vi "Set Object Size Difference.vi"(8 "error in (no error)":errorcluster, 9 "dSize":cluster{"width":i32, "height":i32}, 11 "GObj Refnum":refnum<vi>) -> (0 "error out":errorcluster, 2 "dSize":cluster{"width":i32, "height":i32})   [LabVIEW 2013, in "IObject.lvclass"]
uses:
  IObject.lvclass
  <vilib>/Utility/error.llb/Error Cluster From Error Code.vi
  <vilib>/ErrorRing/Error Ring.xnode
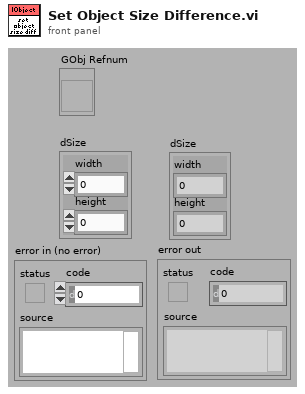
[diagram p1: front panel]
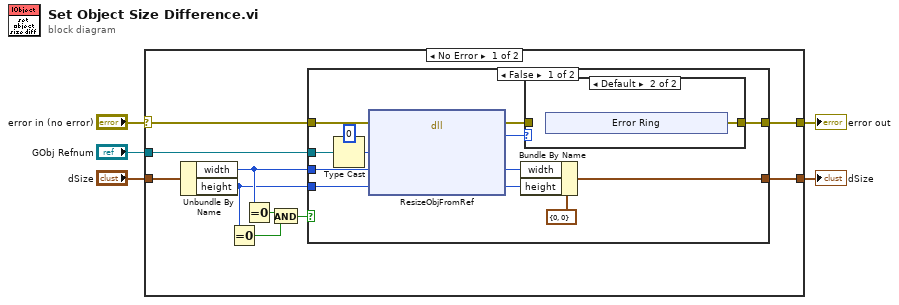
[diagram p0: block diagram]
diagram:
  n1 = case shown="No Error" "error in (no error)" {
    selector: "error in (no error)" -> [w11 w37]
    tunnel: "dSize" -> [w6 _]
    tunnel: [w15 w37] -> w5
    tunnel: "GObj Refnum" -> [w10 _]
    tunnel: [w7 _] -> w1
    frame No Error {
      n2 = Unbundle By Name(w6) -> ("width"=w9:i32, "height"=w8:i32)
      n3 = Equal To 0?(x=w8) -> (x = 0?=w13:bool)
      n4 = Equal To 0?(x=w9) -> (x = 0?=w14:bool)
      n5 = And(x=w14, y=w13) -> (x .and. y?=w12:bool)
      n6 = case shown="False" w12 {
        tunnel: [w28 w36] -> w15
        tunnel: w9 -> [w21 _]
        tunnel: w8 -> [w20 _]
        tunnel: w11 -> [w23 w36]
        tunnel: w10 -> [w27 _]
        tunnel: [w16 _] -> w7
        frame False {
          n7 = Type Cast(type=0, x=w27) -> (*(type *) &x=w24:i32)
          n8 = dll-call lib="LabVIEW" fn="ResizeObjFromRef"(error in=w23, "Reference"=w24, "AddX"=w21, "AddY"=w20) -> (error out=w22:errorcluster, "Bool"=w26:i32, "AddX"=w19:i32, "AddY"=w18:i32)  [unwired: 3 in, 1 out]
          n9 = Bundle By Name(cluster=cluster{"width":i32, "height":i32} {"width"=0, "height"=0} ("dSize"), "width"=w19, "height"=w18) -> (w16:cluster{"width":i32, "height":i32})
          n10 = case shown="Default" w26 {
            tunnel: [w29 w30] -> w28
            tunnel: w22 -> [w29 _]
            frame 0 {
            }
            frame Default {
              n11 = xnode "Error Ring"() -> ("error out"=w30:errorcluster)
            }
          }
        }
        frame True {
        }
      }
    }
    frame Error {
    }
  }
  "error out" <- w5
  "dSize" <- w1
